vi "Generator Test.vi"(8 "error in":errorcluster, 11 "IED Test in":refnum<class "IED Test.lvclass">) -> (0 "error out":errorcluster, 2 "Test Result":T1=enum."Success", 3 "IED Test out":refnum<class "IED Test.lvclass">)   [LabVIEW 2018, in "IED Test Framework.lvlib" / "IED Test.lvclass"]
uses:
  IED Test.lvclass
  C:/Program Files (x86)/National Instruments/LabVIEW 2018/vi.lib/ActorFramework/Actor/Actor.lvclass
  C:/Users/Administrator/Desktop/2018LabVIEW EMS/EMS Generic Actor/EMS Generic/EMS Generic.lvclass
  Controls/Test Result.ctl
  <vilib>/ORNL/CSEISMIC DDS/CSEISMIC DDS Base/Data Types/Controls/DeviceClass Selector.ctl
  Generator Actor/Generator/Generator.lvclass
  C:/Users/Administrator/Desktop/2018LabVIEW EMS/IED Actors/Device DDS Communications Framework/Device DDS Communications/Device DDS Communications.lvclass
  <vilib>/ORNL/CSEISMIC DDS/CSEISMIC DDS Base/CSEISMIC DDS.lvclass/CSEISMIC DDS.ctl
  <vilib>/ORNL/CSEISMIC DDS/CSEISMIC DDS Base/Data Types/Controls/DeviceID.ctl
  <vilib>/ActorFramework/Message Enqueuer/Message Enqueuer.lvclass/Message Enqueuer.ctl
  <vilib>/ORNL/CSEISMIC DDS/CSEISMIC DDS Base/Accessors/Write DDS Reference.vi
  <vilib>/ORNL/CSEISMIC DDS/CSEISMIC DDS Base/Accessors/Read DDS Reference.vi
  <vilib>/ActorFramework/Message Enqueuer/Enqueue.vi
  <vilib>/ORNL/CSEISMIC DDS/DDS Writer/DDS Writer.lvclass
  C:/Program Files (x86)/National Instruments/LabVIEW 2018/vi.lib/ORNL/CSEISMIC DDS/CSEISMIC DDS Base/CSEISMIC DDS.lvclass
  <vilib>/ActorFramework/Stop Msg/Stop Msg.lvclass
  C:/Program Files (x86)/National Instruments/LabVIEW 2018/vi.lib/ActorFramework/Message/Message.lvclass
  <vilib>/ORNL/CSEISMIC DDS/CSEISMIC DDS Base/Error Handler.vi
  <vilib>/ActorFramework/Message Priority Queue/Priority Enqueue.vi
  <vilib>/ORNL/CSEISMIC DDS/CSEISMIC DDS Base/CSEISMIC DDS.lvclass
  Device DDS Communications Framework/Device DDS Communications/Device DDS Communications.lvclass
  <vilib>/ActorFramework/Actor/Actor.lvclass
  EMS Generic Actor/EMS Generic/EMS Generic.lvclass
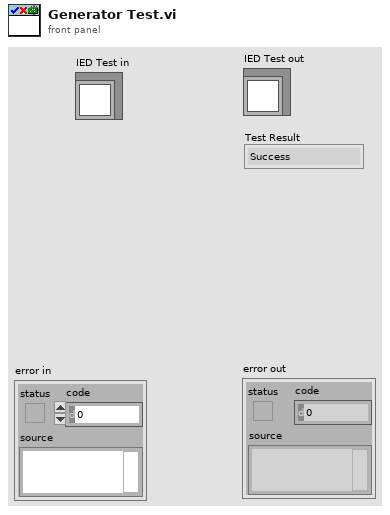
[diagram p1: front panel]
types:
  T1 = typedef "IED Test Framework.lvlib/IED Test.lvclass/Test Result.ctl" = enum16{"Invalid", "Success", "Failure", "Error", "Timeout"}
  T2 = typedef "CSEISMIC DDS.lvlib/CSEISMIC DDS.lvclass/DeviceID.ctl" = string
  T3 = typedef "CSEISMIC DDS.lvlib/CSEISMIC DDS.lvclass/DeviceClass Selector.ctl" = u16
  T4 = typedef "CSEISMIC DDS.lvlib/CSEISMIC DDS.lvclass/Generator_Info.ctl" = cluster{"DeviceID":T2, "Voltage (V)":dbl, "MinimumPower (kVA)":dbl, "EnergyRating (kWh)":dbl, "RampRate (kW/s)":dbl, "MaxPowerFactorLeading":dbl, "MaxPowerFactorLagging":dbl, "EfficiencyCurve":T5, "StartCost":dbl, "FuelCost":dbl, "StartTime (s)":dbl}
  T5 = typedef "CSEISMIC DDS.lvlib/CSEISMIC DDS.lvclass/EfficiencyCurve.ctl" = cluster{"Power (kW)":dbl[], "Efficiency (%)":dbl[]}
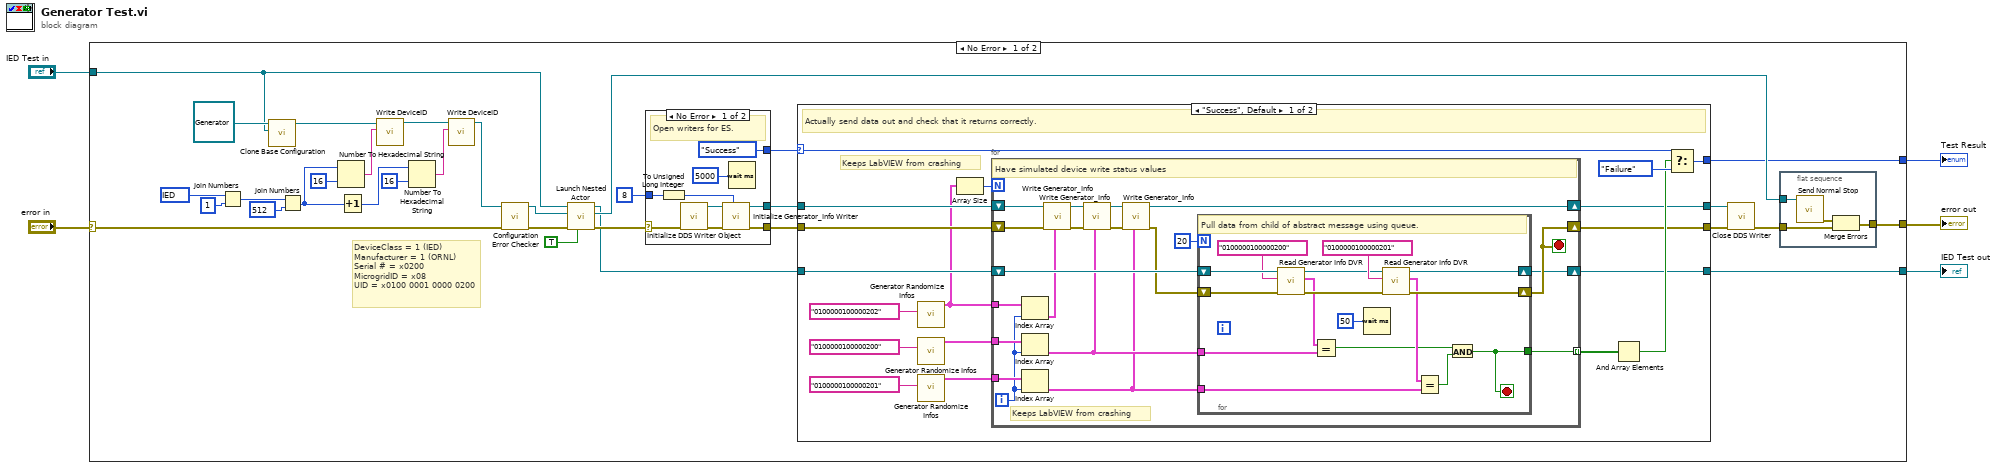
[diagram p0: block diagram]
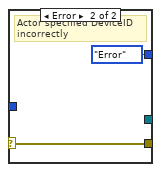
[diagram p3: hidden frame]
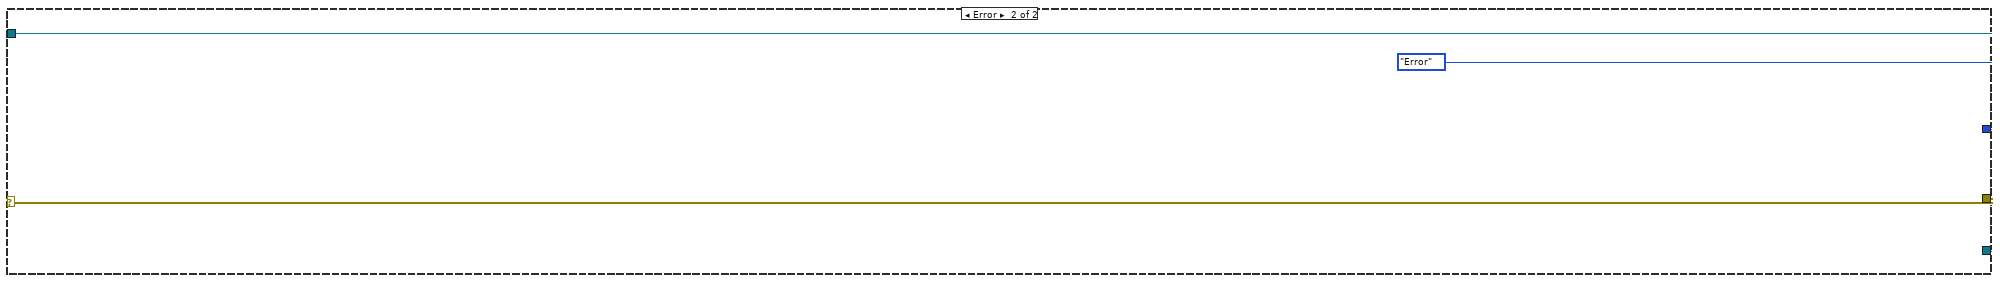
[diagram p4: hidden frame]
diagram:
  n1 = case shown="No Error" "error in" {
    selector: "error in" -> [w33 w113]
    tunnel: [w35 w113] -> w1
    tunnel: [w6 w112] -> w2
    tunnel: "IED Test in" -> [w8 w112]
    tunnel: [w13 Test_Result."Error" ("f")] -> w3
    frame No Error {
      w26 = T3 256 items=["Invalid"=0, "IED"=256, "DER"=512, "Relay"=768, "Meter"=1024, "Load"=1280, "Forecast"=1536, "Price"=1792, "Energy Storage"=513, "PV"=514, "Generator"=515, "Smart Relay"=769, "PCC"=770, "Smart Meter"=1025, "PMU"=1026, "HVAC"=1281] ("DeviceClass")
      # "DeviceClass = 1 (IED)\nManufacturer = 1 (ORNL)\nSerial # = x0200\nMicrogridID = x08\nUID = x0100 0001 0000 0200"
      n2 = Join Numbers(hi=w26, lo=u16 1 ("MicrogridID")) -> ((hi.lo)=w23:u32)
      n3 = call-dynamic "Clone Base Configuration.vi"("Source Object"=w8, "Target Object in"=refnum<class "Generator.lvclass"> refnum ("Generator Actor.lvlib:Generator.lvclass")) -> ("Target Object out"=w9:refnum<class "Generator.lvclass">)  [unwired: 9 in]
      n4 = Join Numbers(hi=w23, lo=u32 512 ("MicrogridID")) -> ((hi.lo)=w28:u64)
      n5 = Number To Hexadecimal String(1:i16 16 ("width (-)"), 2:w28) -> (0:w21:string)
      n6 = Increment(x=w28) -> (x+1=w30:u64)
      n7 = call-dynamic "Write DeviceID.vi"("DeviceID"=w21, "Device DDS Communications in"=w9) -> ("Device DDS Communications out"=w25:refnum<class "Generator.lvclass">)  [unwired: 9 in]
      n8 = Number To Hexadecimal String(1:i16 16 ("width (-)"), 2:w30) -> (0:w31:string)
      n9 = call-dynamic "Write DeviceID.vi"("DeviceID"=w31, "Device DDS Communications in"=w25) -> ("Device DDS Communications out"=w11:refnum<class "Generator.lvclass">)  [unwired: 9 in]
      n10 = call "Configuration Error Checker.vi"("error in"=w33, "Device DDS Communications in"=w11) -> ("error out"=w36:errorcluster, "Device DDS Communications out"=w34:refnum<class "Generator.lvclass">)  [unwired: 8 in]
      n11 = call <vilib>:"Launch Nested Actor.vi"("Open Actor Core front panel? (F)"=TRUE, "error in (no error)"=w36, "Nested Actor"=w34, "Caller Actor in"=w8) -> ("error out"=w19:errorcluster, "Nested Actor's Enqueuer"=w32:refnum<class "Message Enqueuer.lvclass">, "Caller Actor out"=w7:refnum<class "IED Test.lvclass">)  [unwired: 5 in]
      n12 = case shown="No Error" w19 {
        selector: w19 -> [w106 w110]
        tunnel: [w100 w110] -> w16
        tunnel: u32 8 ("domain id") -> [w108 _]
        tunnel: [Test_Result."Success" ("Test Result in") Test_Result."Error" ("Test Result")] -> w18
        tunnel: [w101 _] -> w17
        frame No Error {
          # "Open writers for ES."
          n13 = To Unsigned Long Integer(number=w108) -> (unsigned 32bit integer=w103:u32)
          n14 = call <vilib>:"Initialize DDS Writer Object.vi"("error in"=w106) -> ("error out"=w105:errorcluster, "DDS Writer out"=w104:refnum<class "DDS Writer.lvclass">)  [unwired: 9 in]
          n15 = call <vilib>:"Initialize Generator_Info Writer.vi"("MicrogridID"=w103, "error in"=w105, "DDS Writer in"=w104) -> ("error out"=w100:errorcluster, "DDS Writer out"=w101:refnum<class "DDS Writer.lvclass">)  [unwired: 7 in]
          n16 = Wait (ms)(milliseconds to wait=u32 5000) -> ()  [unwired: 1 out]
        }
        frame Error {
          # "Actor specified DeviceID incorrectly"
        }
      }
      n17 = case shown="\"Success\", Default" w18 {
        selector: w18 -> [w58 w98]
        tunnel: w17 -> [w59 w97]
        tunnel: w7 -> [w53 w96]
        tunnel: w16 -> [w54 w99]
        tunnel: [w56 w98] -> w13
        tunnel: [w52 w99] -> w14
        tunnel: [w50 w97] -> w15
        tunnel: [w42 w96] -> w6
        frame "Success", Default {
          # "Keeps LabVIEW from crashing"
          # "Actually send data out and check that it returns correctly."
          n18 = call "Generator Randomize Infos.vi"("DeviceID"=T2 "0100000100000202" ("(hi.lo)")) -> ("Generator_Info Array out"=w49:T4[])  [unwired: 10 in]
          n19 = call "Generator Randomize Infos.vi"("DeviceID"=T2 "0100000100000200" ("(hi.lo)")) -> ("Generator_Info Array out"=w44:T4[])  [unwired: 10 in]
          n20 = call "Generator Randomize Infos.vi"("DeviceID"=T2 "0100000100000201" ("(hi.lo)")) -> ("Generator_Info Array out"=w45:T4[])  [unwired: 10 in]
          n21 = Array Size(array=w49) -> (size(s)=w51:i32)
          n22 = for {
            N: w51 -> [_]
            shift-right: [w76] -> w50
            shift-left: w59 -> [w79]
            tunnel: w49 -> [w72]
            tunnel: w45 -> [w67]
            tunnel: w44 -> [w68]
            shift-right: [w69] -> w52
            shift-left: w54 -> [w75]
            shift-right: [w61] -> w42
            shift-left: w53 -> [w71]
            tunnel: [w60] -> w43 mode=indexing
            i -> [w65]
            stop <- w69 stop-if-true
            # "Keeps LabVIEW from crashing"
            # "Have simulated device write status values"
            n23 = Index Array(array=w72, index=w65) -> (element=w64:T4)
            n24 = Index Array(array=w68, index=w65) -> (element=w63:T4)
            n25 = Index Array(array=w67, index=w65) -> (element=w62:T4)
            n26 = call <vilib>:"Write Generator_Info.vi"("Generator_Info"=w64, "error in"=w75, "DDS Writer in"=w79) -> ("error out"=w74:errorcluster, "DDS Writer out"=w78:refnum<class "DDS Writer.lvclass">)  [unwired: 7 in]
            n27 = call <vilib>:"Write Generator_Info.vi"("Generator_Info"=w63, "error in"=w74, "DDS Writer in"=w78) -> ("error out"=w73:errorcluster, "DDS Writer out"=w77:refnum<class "DDS Writer.lvclass">)  [unwired: 7 in]
            n28 = call <vilib>:"Write Generator_Info.vi"("Generator_Info"=w62, "error in"=w73, "DDS Writer in"=w77) -> ("error out"=w70:errorcluster, "DDS Writer out"=w76:refnum<class "DDS Writer.lvclass">)  [unwired: 7 in]
            n29 = for {
              N: 20 -> [_]
              shift-right: [w88] -> w69
              shift-left: w70 -> [w94]
              shift-right: [w89] -> w61
              shift-left: w71 -> [w95]
              tunnel: w63 -> [w87]
              tunnel: w62 -> [w84]
              tunnel: [w81] -> w60
              stop <- w81 stop-if-true
              # "Pull data from child of abstract message using queue."
              n30 = call "Read Generator Info DVR.vi"("error in"=w94, "DeviceID"=T2 "0100000100000200" ("(hi.lo)"), "EMS Generic in"=w95) -> ("error out"=w90:errorcluster, "Generator_Info"=w86:T4, "EMS Generic out"=w91:refnum<class "IED Test.lvclass">)  [unwired: 5 in, 1 out]
              n31 = Equal?(x=w86, y=w87) -> (x = y?=w83:bool)
              n32 = Wait (ms)(milliseconds to wait=u32 50) -> ()  [unwired: 1 out]
              n33 = call "Read Generator Info DVR.vi"("error in"=w90, "DeviceID"=T2 "0100000100000201" ("(hi.lo)"), "EMS Generic in"=w91) -> ("error out"=w88:errorcluster, "Generator_Info"=w85:T4, "EMS Generic out"=w89:refnum<class "IED Test.lvclass">)  [unwired: 5 in, 1 out]
              n34 = Equal?(x=w85, y=w84) -> (x = y?=w82:bool)
              n35 = And(x=w83, y=w82) -> (x .and. y?=w81:bool)
            }
          }
          n36 = And Array Elements(Boolean array=w43) -> (logical AND=w55:bool)
          n37 = Select(t=w58, s=w55, f=Test_Result."Failure") -> (s? t:f=w56:T1)
        }
        frame "Error" {
        }
      }
      n38 = call <vilib>:"Close DDS Writer.vi"("error in"=w14, "DDS Writer in"=w15) -> ("error out"=w12:errorcluster)  [unwired: 9 in]
      n39 = flat-sequence {
        tunnel: w32 -> [w41]
        tunnel: [w39] -> w35
        tunnel: w12 -> [w38]
        frame #0 {
          n40 = call <vilib>:"Send Normal Stop.vi"("Message Enqueuer"=w41) -> ("error out"=w40:errorcluster)  [unwired: 10 in]
          n41 = Merge Errors(w40, w38) -> (w39:errorcluster)
        }
      }
    }
    frame Error {
    }
  }
  "error out" <- w1
  "IED Test out" <- w2
  "Test Result" <- w3
